vi "set Defaults.vi"(0 "Session in":refnum<class "SLSC Session.lvclass">, 11 "error in":errorcluster) -> (4 "Session out":refnum<class "SLSC Session.lvclass">, 15 "error out":errorcluster)   [LabVIEW 2015, in "SLSC Switch.lvlib" / "SLSC Session.lvclass"]
uses:
  SLSC Session.lvclass
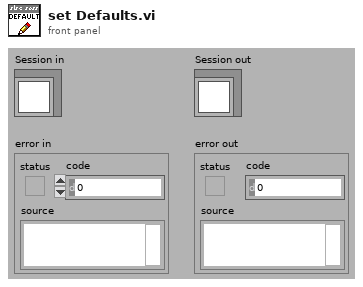
[diagram p1: front panel]
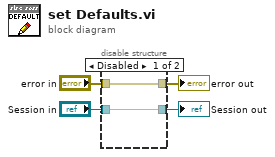
[diagram p0: block diagram]
diagram:
  n1 = disable-structure shown="Disabled" {
    disable-tunnel: "Session in" -> [w5 w8]
    disable-tunnel: [w5 w8] -> w3
    disable-tunnel: "error in" -> [w6 w7]
    disable-tunnel: [w6 w7] -> w4
    frame Disabled {
    }
    frame Enabled {
    }
  }
  "error out" <- w4
  "Session out" <- w3
